vi "Main_SAIDD-Steffen’s MacBook Pro.vi"() -> ()   [LabVIEW 2018]
uses:
  <extravilib>/ChannelInstances/Tag-bool/Read With Abort.vi
  <extravilib>/ChannelInstances/Tag-bool/Write With Abort.vi
  <vilib>/myRIO/Common/Instrument Driver Framework/myRIO v1.0/UART/vis/myRIO v1.0 Close UART.vi
  <vilib>/Utility/error.llb/Error Cluster From Error Code.vi
  <vilib>/myRIO/Common/Instrument Driver Framework/myRIO v1.0/PWM/vis/myRIO v1.0 Write PWM.vi
  <vilib>/myRIO/Common/Instrument Driver Framework/myRIO v1.0/DIO/vis/myRIO v1.0 Write DIO.vi
  <extravilib>/ChannelInstances/Tag-bool/Instantiate.vi
  <extravilib>/ChannelInstances/Tag-bool/EndpointRead.vi
  <extravilib>/ChannelInstances/Tag-bool/Endpoint.vi
  <vilib>/myRIO/Common/Instrument Driver Framework/Utilities/vis/FPGA Ref Manager.vi
  <vilib>/myRIO/Common/Instrument Driver Framework/myRIO v1.0/myRIO v1.0 Reset FPGA.vi
  <vilib>/myRIO/Common/Instrument Driver Framework/myRIO v1.0/IRQ/vis/myRIO v1.0 IRQ Info FGV.vi
  <vilib>/myRIO/Common/Instrument Driver Framework/myRIO v1.0/IRQ/vis/myRIO v1.0 Timer IRQ Info FGV.vi
  <vilib>/myRIO/Common/Instrument Driver Framework/myRIO v1.0/IRQ/vis/myRIO v1.0 ISR Agent.vi
  <extravilib>/ChannelInstances/Tag-bool.lvlib
  <vilib>/myRIO/Instrument Drivers/Onboard IO/DIO/DIO.lvlib
  <vilib>/myRIO/Instrument Drivers/Onboard IO/PWM/PWM.lvlib
  <vilib>/myRIO/Instrument Drivers/Utilities/Utilities.lvlib
panel:
  in  "Beacon - test":bool
  in  "Grounded threshold":dbl=1.7 format="%#_13g"
  in  "QR - test":bool
  in  "Enable Triangle Wobble":bool=TRUE
  in  "Antal iterationer pr. stepper":i32=800
  in  "Stop":bool
  out "Measured current":dbl
  out "Ammeter measurement":dbl(graph)
  out "Duty Cycle":dbl
  out "Mean 200":dbl format="%0.2f"
  out "Battery left (%)":dbl
  in  "Drill - Frequency [Hz]":dbl=200.0
  in  "Stepper frekvens ned":dbl=120.0
  in  "Ingen modstand ned upper threshold":dbl=2750.0
  out "ALL TOP":bool
  out "ALL BOTTOM":bool
  in  "Resistance - Threshold Upper":dbl=3100.0
  in  "Resistance Threshold Lower":dbl=3025.0
  out "Process":T1(ring)
  in  "State":T1(ring)
  in  "high cutoff freq: fh":dbl=900.0
  in  "Radius":dbl=0.005 format="%#_13g"
  in  "Filter?":bool=TRUE
  out "RollDetection - Alarm":bool
types:
  T1 = enum16{"State 0 - Default", "State 1 - Go down", "State 2 - Go up", "State 3 - Triangle Wobble"}
  T2 = typedef "DIO.lvlib/DIO Reference.ctl" = cluster{"myRIO Reference":T3, "DIO Channels List":T7}
  T3 = typedef "myRIO Generic Hardware Reference.ctl" = cluster{"myRIO Model":T4, "myRIO Hardware Reference":T5}
  T4 = typedef "Hardware Version Enum.ctl" = enum16{"Unknown", "myRIO-1900", "myRIO-1950", "roboRIO", "NI ELVIS RIO CM", "ELVIS III"}
  T5 = typedef "myRIO v1.0 Reference.ctl" = cluster{"Generic FPGA Reference":T6, "Allow multiple opens":bool}
  T6 = typedef "Generic FPGA Reference.ctl" = refnum<k20>
  T7 = typedef "DIO Channels List.ctl" = T8[]
  T8 = typedef "DIO Channels Enum.ctl" = enum16{"Not Connected", "C/DIO0", "C/DIO1", "C/DIO2", "C/DIO3", "C/DIO4", "C/DIO5", "C/DIO6", "C/DIO7", "A/DIO0", "A/DIO1", "A/DIO2", "A/DIO3", "A/DIO4", "A/DIO5", "A/DIO6", "A/DIO7", "A/DIO8", "A/DIO9", "A/DIO10", "A/DIO11", "A/DIO12", "A/DIO13", "A/DIO14", "A/DIO15", "A/DIO16", "A/DIO17", "A/DIO18", "A/DIO19", "B/DIO0", "B/DIO1", "B/DIO2", "B/DIO3", "B/DIO4", "B/DIO5", "B/DIO6", "B/DIO7", "B/DIO8", "B/DIO9", "B/DIO10", "B/DIO11", "B/DIO12", "B/DIO13", "B/DIO14", "B/DIO15", "B/DIO16", "B/DIO17", "B/DIO18", "B/DIO19", "LED0", "LED1", "LED2", "LED3", "Button0", "DIO/DIO0", "DIO/DIO1", "DIO/DIO2", "DIO/DIO3", "DIO/DIO4", "DIO/DIO5", "DIO/DIO6", "DIO/DIO7", "DIO/DIO8", "DIO/DIO9", "SPI/CS0", "SPI/CS1", "SPI/CS2", "SPI/CS3", "LED RADIO (Green)", "LED RADIO (Red)", "LED COMM (Green)", "LED COMM (Red)", "LED MODE (Green)", "LED MODE (Red)"}
  T9 = typedef "PWM.lvlib/PWM Reference.ctl" = cluster{"myRIO Reference":T3, "PWM Channels Enum":T10, "PWM Configuration":T11}
  T10 = typedef "PWM Channels Enum.ctl" = enum16{"Not Connected", "C/PWM0", "C/PWM1", "A/PWM0", "A/PWM1", "A/PWM2", "A/PWM3", "A/PWM4", "A/PWM5", "A/PWM6", "A/PWM7", "A/PWM8", "A/PWM9", "A/PWM10", "A/PWM11", "A/PWM12", "A/PWM13", "A/PWM14", "A/PWM15", "A/PWM16", "A/PWM17", "A/PWM18", "A/PWM19", "B/PWM0", "B/PWM1", "B/PWM2", "B/PWM3", "B/PWM4", "B/PWM5", "B/PWM6", "B/PWM7", "B/PWM8", "B/PWM9", "B/PWM10", "B/PWM11", "B/PWM12", "B/PWM13", "B/PWM14", "B/PWM15", "B/PWM16", "B/PWM17", "B/PWM18", "B/PWM19", "PWM/PWM0", "PWM/PWM1", "PWM/PWM2", "PWM/PWM3", "PWM/PWM4", "PWM/PWM5", "PWM/PWM6", "PWM/PWM7", "PWM/PWM8", "PWM/PWM9"}
  T11 = typedef "PWM.lvlib/PWM Configuration.ctl" = cluster{"Frequency":dbl, "Duty Cycle":dbl}
  T12 = typedef "Accelerometer.lvlib/Accelerometer Reference.ctl" = cluster{"myRIO Reference":T3, "Accelerometer Channels List":T13, "LSB Weight":dbl}
  T13 = typedef "Accelerometer Channels List.ctl" = T14[]
  T14 = typedef "Accelerometer Channels Enum.ctl" = enum16{"Not Connected", "X-Axis", "Y-Axis", "Z-Axis"}
  T15 = typedef "AI.lvlib/AI Reference.ctl" = cluster{"myRIO Reference":T3, "AI Channels List":T16, "AI Scaling Constants List":T18}
  T16 = typedef "AI Channels List.ctl" = T17[]
  T17 = typedef "AI Channels Enum.ctl" = enum16{"Not Connected", "AudioIn/Left", "AudioIn/Right", "C/AI0", "C/AI1", "A/AI0", "A/AI1", "A/AI2", "A/AI3", "A/AI4", "A/AI5", "A/AI6", "A/AI7", "B/AI0", "B/AI1", "B/AI2", "B/AI3", "B/AI4", "B/AI5", "B/AI6", "B/AI7", "AI/AI0", "AI/AI1", "AI/AI2", "AI/AI3", "A/AI0 (DIFF)", "A/AI1 (DIFF)", "A/AI2 (DIFF)", "A/AI3 (DIFF)", "B/AI0 (DIFF)", "B/AI1 (DIFF)", "B/AI2 (DIFF)", "B/AI3 (DIFF)"}
  T18 = typedef "Analog Scaling Constants List.ctl" = T19[]
  T19 = typedef "Analog Scaling Constants.ctl" = cluster{"LSB Weight (Volts)":dbl, "Offset (Volts)":dbl, "Signed?":bool}
  T20 = typedef "SPI.lvlib/SPI Reference.ctl" = cluster{"myRIO Reference":T3, "SPI Channels Enum":T21, "SPI Configuration":T22}
  T21 = typedef "SPI Channels Enum.ctl" = enum16{"Not Connected", "A/SPI", "B/SPI", "SPI/SPI"}
  T22 = typedef "SPI.lvlib/SPI Configuration.ctl" = cluster{"Frequency [Hz]":dbl, "Clock Phase":T23, "Clock Polarity":T24, "Data Direction":T25, "Frame Length":T26}
  T23 = typedef "SPI Clock Phase.ctl" = enum8{"Leading", "Trailing"}
  T24 = typedef "SPI Clock Polarity.ctl" = enum8{"Low", "High"}
  T25 = typedef "SPI Data Direction.ctl" = enum8{"Most significant bit first", "Least significant bit first"}
  T26 = typedef "SPI Frame Length.ctl" = u8
  T27 = cluster{"B/DIO0 - Stepper Direction":T2, "B/DIO1 - Stepper1 Enable":T2, "B/DIO2 - Stepper2 Enable":T2, "B/DIO3 - Stepper3 Enable":T2, "B/DIO4 - Endstop Stepper1 Top":T2, "B/DIO11 - Endstop Stepper1 Bund":T2, "B/DIO12 - Endstop Stepper2 Top":T2, "B/DIO13 - Endstop Stepper2 Bund":T2, "B/DIO14 - Endstop Stepper3 Top":T2, "B/DIO15 - Endstop Stepper3 Bund":T2, "Deleted - A/DIO0 - Cooler":T2, "A/DIO1 - Beacon drop (dio1)":T2, "A/DIO2 - Beacon drop (dio0)":T2, "A/DIO3 - QuickRelease (dio1)":T2, "A/DIO4 - QuickRelease (dio0)":T2, "Deleted - A/DIO11 - LiDAR SPI CS":T2, "B/PWM0 - Stepper":T9, "B/PWM1 - Drill":T9, "Deleted - A/PWM0 - Servo_Roll":T9, "Deleted - A/PWM1 - Servo_Yaw":T9, "Acc. X-axis":T12, "Acc. Y-axis":T12, "B/AI0 - Drone Grounded S1 - F3":T15, "A/AI0 - QuickRelease S4 - F4":T15, "B/AI2 - Beacon Drop S5 - F5":T15, "B/AI3 - Begin drilling S3 - F6":T15, "B/AI1 - Gimbal Seach S8 - F8":T15, "Deleted - A/AI1 - Beacon Wiper":T15, "A/AI2 - QuickRelease Wiper":T15, "A/AI3 - Drill Current":T15, "Deleted - A/SPI - LiDAR":T20, "B/UART - XBee":refnum<visa-resource-name>, "Deleted - A/UART - A3 GPS":refnum<visa-resource-name>, "RIO Flashing LEDs":T2}
  T28 = typedef "Tag-bool.lvlib/))Channel.ctl" = refnum<queue>
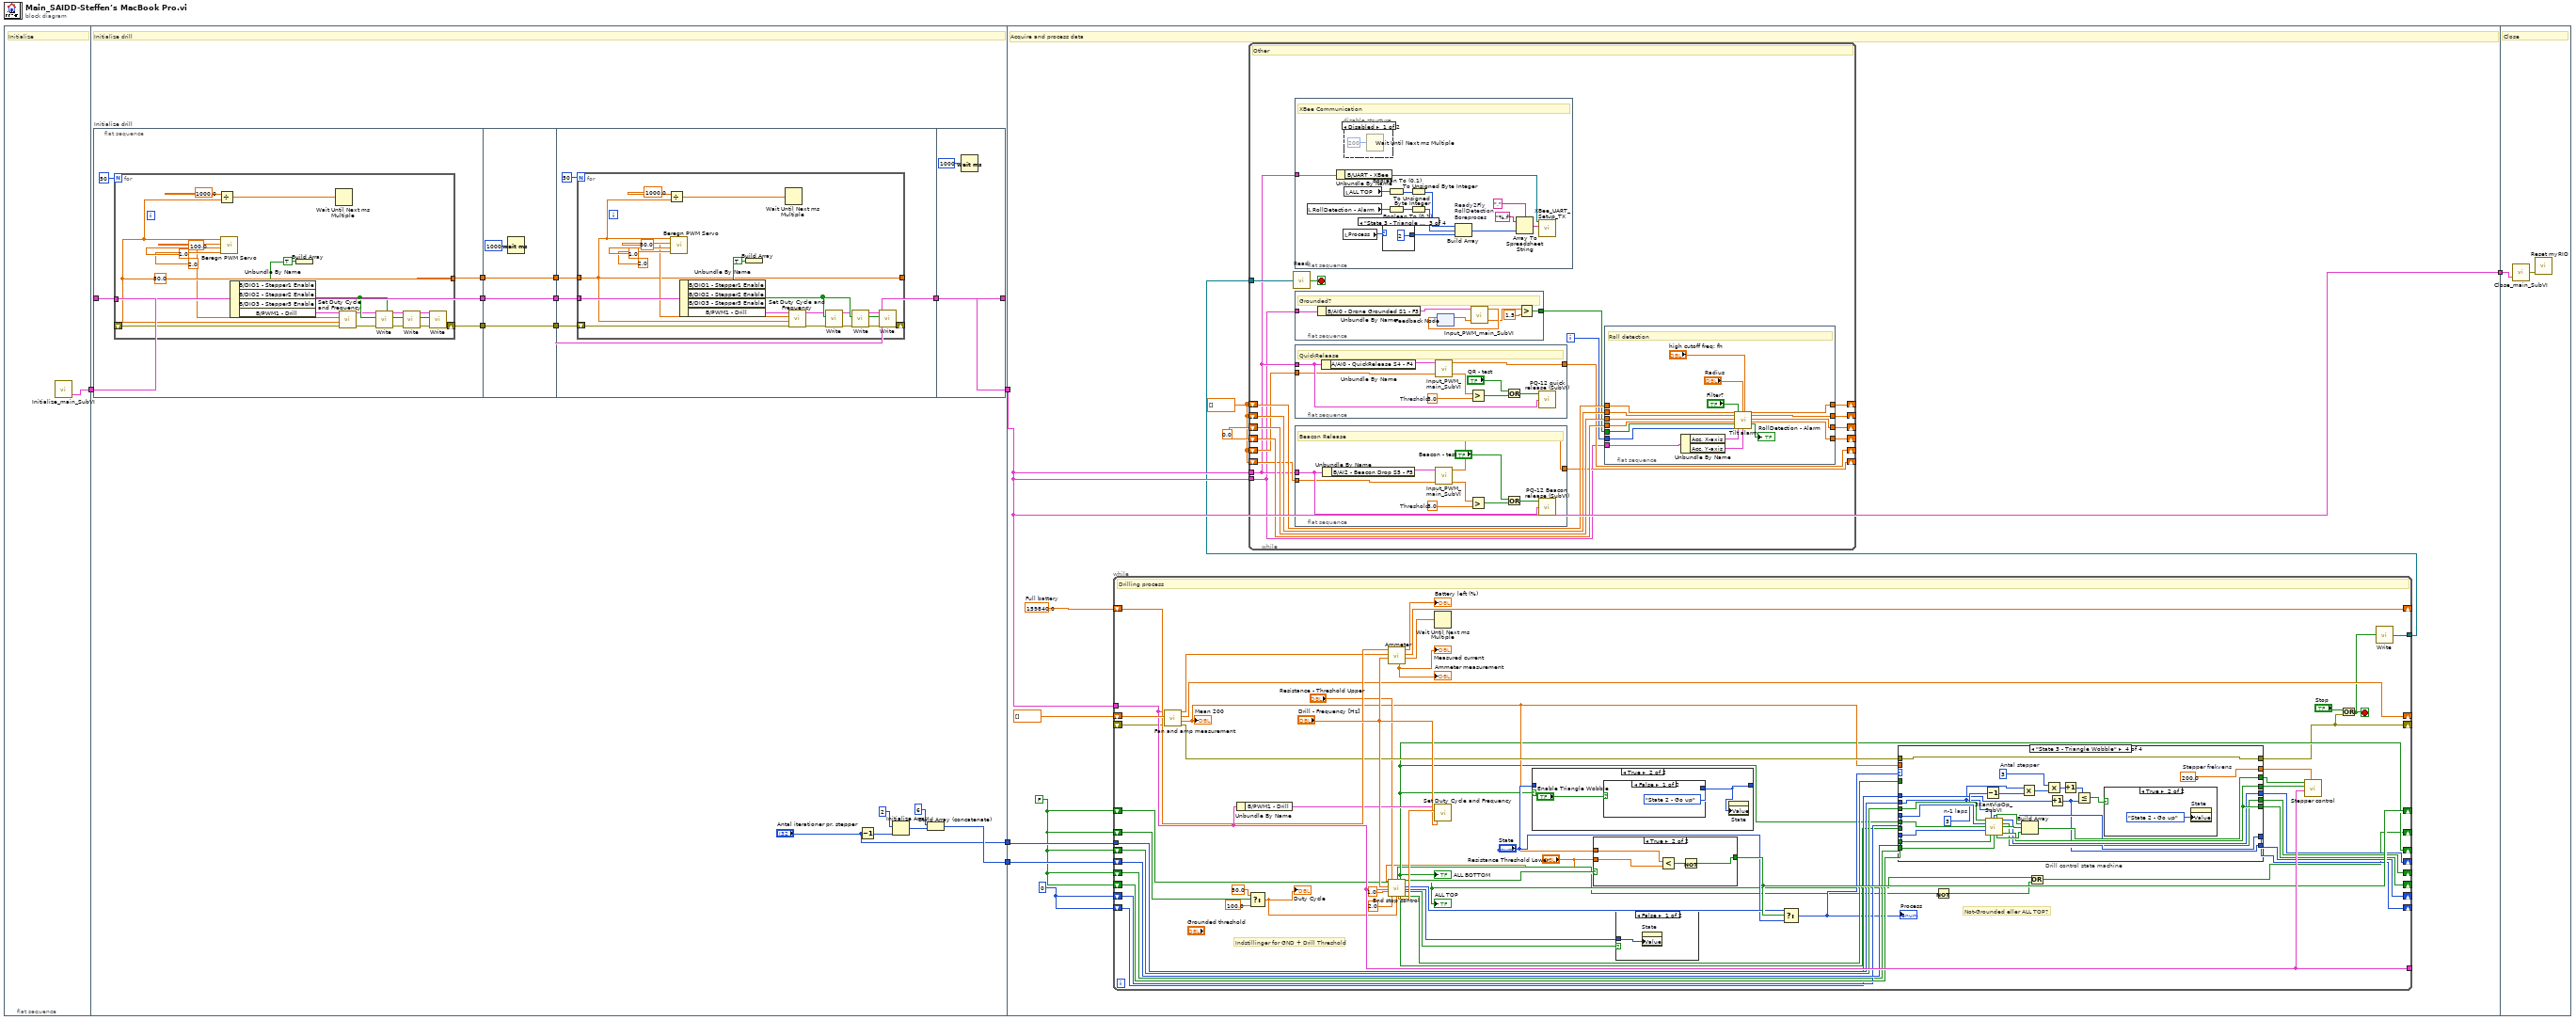
[diagram p0: block diagram]
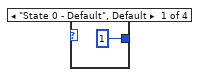
[diagram p3: hidden frame]
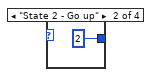
[diagram p4: hidden frame]
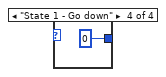
[diagram p5: hidden frame]
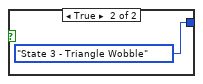
[diagram p8: hidden frame]
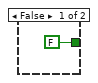
[diagram p9: hidden frame]
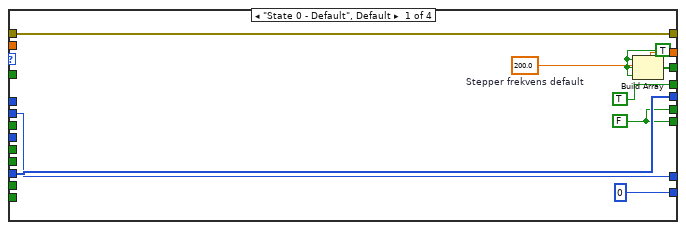
[diagram p10: hidden frame]
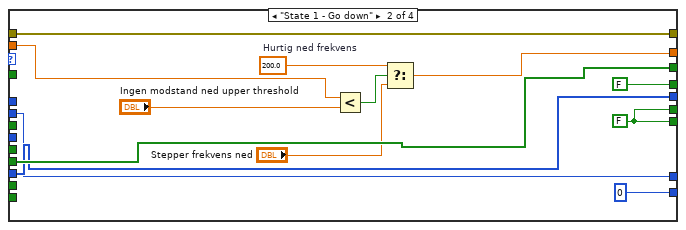
[diagram p11: hidden frame]
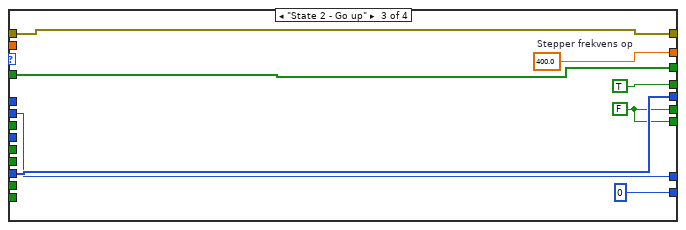
[diagram p12: hidden frame]
diagram:
  n1 = flat-sequence {
    tunnel: [w6] -> w4
    tunnel: w4 -> [w21]
    tunnel: [w18] -> w3
    tunnel: ["Antal iterationer pr. stepper"] -> w2
    tunnel: [w12] -> w1
    tunnel: w3 -> [w76]
    tunnel: [w76] -> w5
    tunnel: w2 -> [w79]
    tunnel: w1 -> [w78]
    tunnel: w5 -> [w289]
    frame #0 {
      # "Initialize"
      n2 = call "Initialize_main_SubVI.vi"() -> ("output cluster"=w6:T27)  [unwired: 2 in, 1 out]
    }
    frame #1 {
      # "Initialize drill"
      n3 = flat-sequence "Initialize drill" {
        tunnel: w21 -> [w25]
        tunnel: [w25] -> w20
        tunnel: [w24] -> w9
        tunnel: [w23] -> w7
        tunnel: w20 -> [w48]
        tunnel: [w48] -> w19
        tunnel: [w46] -> w10
        tunnel: w9 -> [w46]
        tunnel: [w45] -> w8
        tunnel: w7 -> [w45]
        tunnel: w19 -> [w52]
        tunnel: [w52] -> w17
        tunnel: w10 -> [w51]
        tunnel: w8 -> [w50]
        tunnel: [w73] -> w18
        tunnel: w17 -> [w73]
        frame #0 {
          n4 = for {
            N: 50 -> [_]
            tunnel: [w39] -> w24
            shift-right: [w32] -> w23
            shift-left: _ -> [w41]
            tunnel: w25 -> [w37]
            w39 = 50.0 ("Frequency [Hz]")
            n5 = Divide(x=1000.0, y=w39) -> (x/y=w40:dbl)
            n6 = call "Beregn PWM Servo.vi"("Max (ms puls bredde)"=2.0, "Min (ms puls bredde)"=1.0, "Duty Cycle"=100.0, "Frekvens"=w39) -> ("Output Dutycycle til PWM Servo"=w26:dbl)  [unwired: 7 in]
            n7 = Unbundle By Name(w37) -> ("B/DIO1 - Stepper1 Enable"=w27:T2, "B/DIO2 - Stepper2 Enable"=w28:T2, "B/DIO3 - Stepper3 Enable"=w29:T2, "B/PWM1 - Drill"=w31:T9)
            n8 = Build Array(TRUE) -> (w30:bool[])
            n9 = Wait Until Next ms Multiple(millisecond multiple=w40) -> ()  [unwired: 1 out]
            n10 = call <vilib>:"Set Duty Cycle and Frequency.vi"("error in (no error)"=w41, "Frequency [Hz]"=w39, "Duty Cycle"=w26, "PWM Ref In"=w31) -> ("error out"=w35:errorcluster)  [unwired: 5 in, 1 out]
            n11 = call <extravilib>:"Write.vi"("error in (no error)"=w35, "Values"=w30, "DIO Ref In"=w29) -> ("error out"=w34:errorcluster)  [unwired: 6 in, 1 out]
            n12 = call <extravilib>:"Write.vi"("error in (no error)"=w34, "Values"=w30, "DIO Ref In"=w28) -> ("error out"=w33:errorcluster)  [unwired: 6 in, 1 out]
            n13 = call <extravilib>:"Write.vi"("error in (no error)"=w33, "Values"=w30, "DIO Ref In"=w27) -> ("error out"=w32:errorcluster)  [unwired: 6 in, 1 out]
          }
        }
        frame #1 {
          n14 = Wait (ms)(milliseconds to wait=u32 1000) -> ()  [unwired: 1 out]
        }
        frame #2 {
          n15 = for {
            N: 50 -> [_]
            tunnel: [w53] -> _
            shift-right: [w60] -> _
            shift-left: w50 -> [w68]
            tunnel: w52 -> [w65]
            tunnel: w51 -> [w53]
            n16 = Divide(x=1000.0, y=w53) -> (x/y=w67:dbl)
            n17 = call "Beregn PWM Servo.vi"("Max (ms puls bredde)"=2.0, "Min (ms puls bredde)"=1.0, "Duty Cycle"=50.0, "Frekvens"=w53) -> ("Output Dutycycle til PWM Servo"=w54:dbl)  [unwired: 7 in]
            n18 = Unbundle By Name(w65) -> ("B/DIO1 - Stepper1 Enable"=w55:T2, "B/DIO2 - Stepper2 Enable"=w56:T2, "B/DIO3 - Stepper3 Enable"=w57:T2, "B/PWM1 - Drill"=w59:T9)
            n19 = Build Array(TRUE) -> (w58:bool[])
            n20 = Wait Until Next ms Multiple(millisecond multiple=w67) -> ()  [unwired: 1 out]
            n21 = call <vilib>:"Set Duty Cycle and Frequency.vi"("error in (no error)"=w68, "Frequency [Hz]"=w53, "Duty Cycle"=w54, "PWM Ref In"=w59) -> ("error out"=w63:errorcluster)  [unwired: 5 in, 1 out]
            n22 = call <extravilib>:"Write.vi"("error in (no error)"=w63, "Values"=w58, "DIO Ref In"=w57) -> ("error out"=w62:errorcluster)  [unwired: 6 in, 1 out]
            n23 = call <extravilib>:"Write.vi"("error in (no error)"=w62, "Values"=w58, "DIO Ref In"=w56) -> ("error out"=w61:errorcluster)  [unwired: 6 in, 1 out]
            n24 = call <extravilib>:"Write.vi"("error in (no error)"=w61, "Values"=w58, "DIO Ref In"=w55) -> ("error out"=w60:errorcluster)  [unwired: 6 in, 1 out]
          }
        }
        frame #3 {
          n25 = Wait (ms)(milliseconds to wait=u32 1000) -> ()  [unwired: 1 out]
        }
      }
      n26 = Decrement(x="Antal iterationer pr. stepper") -> (x-1=w16:i32)
      n27 = Initialize Array(2, w16) -> (w15:i32[])
      n28 = Build Array (concatenate)(6, w15) -> (w12:i32[])
    }
    frame #2 {
      w80 = 0.0 ("X-Stored-Shift-out")
      w81 = 0 ("Loops shift out")
      w77 = FALSE ("t")
      w83 = 159840.0  # Full battery
      w74 = dbl[] [] ("X-Array-Shift-out")
      # "Acquire and process data"
      n29 = while {
        shift-right: [w171] -> _
        shift-left: _ -> [w203]
        shift-right: [w175] -> _
        shift-left: dbl[] [] -> [w217]
        shift-right: [w213] -> _
        shift-left: w83 -> [w214]
        tunnel: w76 -> [w209]
        tunnel: [w209] -> _
        shift-right: [w205] -> _
        shift-left: w77 -> [w204]
        shift-right: [w168] -> _
        shift-left: w77 -> [w201]
        shift-right: [w199] -> _
        shift-left: w77 -> [w198]
        shift-right: [w197] -> _
        shift-left: w78 -> [w196]
        tunnel: w79 -> [w190]
        shift-right: [w194] -> _
        shift-left: w81 -> [w195]
        shift-right: [w193] -> _
        shift-left: w77 -> [w192]
        shift-right: [w173] -> _
        shift-left: w77 -> [w191]
        shift-right: [w188] -> _
        shift-left: w81 -> [w189]
        tunnel: [w164] -> w75
        stop <- w165 stop-if-true
        # "Not-Grounded eller ALL TOP?"
        # "Indstillinger for GND + Drill Threshold"
        # "Drilling process"
        n30 = call "Fan and amp measurement.vi"("error in (no error)"=w203, "Array in"=w217, "output cluster"=w209) -> ("error out"=w210:errorcluster, "Mean out"=w174:dbl, "Array out"=w175:dbl[], "dbl Scaled Value"=w207:dbl)  [unwired: 5 in]
        "Mean 200" <- w174
        n31 = Unbundle By Name(w209) -> ("B/PWM1 - Drill"=w211:T9)
        n32 = Select(t=50.0, s=w201, f=100.0 ("upper limit")) -> (s? t:f=w172:dbl)
        "Duty Cycle" <- w172
        n33 = call "Ammeter.vi"("Bor - Frequency [Hz]"="Drill - Frequency [Hz]", "Måling ammeter"=w207, "Sum batteri shift in"=w214) -> ("Wait ud"=w206:dbl, "Sum batteri shift ud"=w213:dbl, "Batteri tilbage (%)"=→"Battery left (%)":dbl, "Målt ampere"=→"Measured current" →"Ammeter measurement":dbl)  [unwired: 5 in]
        n34 = call "End stop control.vi"("Threshold Lower"="Resistance Threshold Lower", "t"=w204, "Bor - Frequency [Hz]"="Drill - Frequency [Hz]", "output cluster"=w209, "Min (ms puls bredde)"=1.0, "Threshold Upper"="Resistance - Threshold Upper", "Max (ms puls bredde)"=2.0, "Bor - Duty Cycle"=w172) -> ("Grounded?"=w166:bool, "Output Dutycycle \nPWM"=w216:dbl, "ALL BOTTOM"=w173:bool, "Bottom Array"=w185:bool[], "Boolean 2"=w182:bool, "ALL TOP"=w169:bool, "Enum 2"=w181:T1, "Enum"=w178:T1, "Boolean"=w179:bool, "Top Array"=w184:bool[])  [unwired: 8 in, 2 out]
        "ALL TOP" <- w169
        "ALL BOTTOM" <- w173
        n35 = Wait Until Next ms Multiple(millisecond multiple=w206) -> ()  [unwired: 1 out]
        n36 = call <vilib>:"Set Duty Cycle and Frequency.vi"("Frequency [Hz]"="Drill - Frequency [Hz]", "Duty Cycle"=w216, "PWM Ref In"=w211) -> ()  [unwired: 6 in, 2 out]
        n37 = case shown="True" w173 {
          tunnel: [w221 w222] -> _
          tunnel: "State" -> [w221 _]
          frame False {
          }
          frame True {
            n38 = case shown="False" "Enable Triangle Wobble" {
              tunnel: [T1."State 2 - Go up" ("Enum") T1."State 3 - Triangle Wobble" ("Enum")] -> w222
              frame False {
              }
              frame True {
              }
            }
            n39 = property on="State" class="Enum (strict)"("Value"=w222) -> ()  [unwired: 2 in, 2 out]
          }
        }
        n40 = case shown="True" w182 {
          tunnel: [FALSE w228] -> w205
          tunnel: w174 -> [_ w230]
          tunnel: "Resistance Threshold Lower" -> [_ w227]
          frame False {
          }
          frame True {
            n41 = Less?(x=w230, y=w227) -> (x < y?=w229:bool)
            n42 = Not(x=w229) -> (.not. x?=w228:bool)
          }
        }
        n43 = case shown="False" w179 {
          tunnel: w178 -> [w220 _]
          frame False {
            n44 = property on="State" class="Enum (strict)"("Value"=w220) -> ()  [unwired: 2 in, 2 out]
          }
          frame True {
          }
        }
        n45 = Select(t=w181, s=w205, f="State") -> (s? t:f=w177:T1)
        "Process" <- w177
        n46 = case "Drill control state machine" shown="\"State 3 - Triangle Wobble\"" w177 {
          tunnel: [w237 w252 w260 w281] -> w176
          tunnel: w185 -> [_ w252 _ _]
          tunnel: w184 -> [_ _ w260 _]
          tunnel: [TRUE FALSE TRUE w280] -> w208
          tunnel: w210 -> [w236 w250 w258 w285]
          tunnel: [w236 w250 w258 w285] -> w171
          tunnel: [w235 w247 w257 w286] -> w202
          tunnel: w174 -> [_ w244 _ _]
          tunnel: [w232 w241 w254 w280] -> w199
          tunnel: w198 -> [_ _ _ w279]
          tunnel: [w234 w243 w256 w278] -> w197
          tunnel: w196 -> [w234 w243 w256 w277]
          tunnel: w190 -> [w233 w242 w255 w267]
          tunnel: w195 -> [_ _ _ w276]
          tunnel: [w233 w242 w255 w275] -> w194
          tunnel: [w232 w241 w254 w274] -> w193
          tunnel: w192 -> [_ _ _ w273]
          tunnel: w191 -> [_ _ _ w272]
          tunnel: w173 -> [_ _ _ w270]
          tunnel: w189 -> [_ _ _ w269]
          tunnel: [0 0 0 w264] -> w188
          frame "State 0 - Default", Default {
            w232 = FALSE
            w235 = 200.0  # Stepper frekvens default
            w238 = TRUE
            n47 = Build Array(w238, w238, w238) -> (w237:bool[])
          }
          frame "State 1 - Go down" {
            w241 = FALSE
            w246 = 200.0  # Hurtig ned frekvens
            n48 = Less?(x=w244, y="Ingen modstand ned upper threshold") -> (x < y?=w249:bool)
            n49 = Select(t=w246, s=w249, f="Stepper frekvens ned") -> (s? t:f=w247:dbl)
          }
          frame "State 2 - Go up" {
            w254 = FALSE
            w257 = 400.0  # Stepper frekvens op
          }
          frame "State 3 - Triangle Wobble" {
            w265 = 3  # Antal stepper
            w271 = 3  # n-1 laps
            w286 = 200.0  # Stepper frekvens
            n50 = Decrement(x=w271) -> (x-1=w268:i32)
            n51 = call "3KantVipOp_SubVI.vi"("Shift 1 in"=w272, "Antal iterationer pr. stepper"=w267, "Loops shift in"=w276, "BUND!"=w270, "Index step array shift in"=w277, "Shift 2 in"=w273, "Shift 3 in"=w279) -> ("Loops shift out"=w275:i32, "Enable 1"=w282:bool, "Index step array shift ud"=w278:i32[], "Shift 2 ud"=w274:bool, "Enable 2"=w283:bool, "Enable 3"=w284:bool, "Direction"=w280:bool)  [unwired: 1 in, 1 out]
            n52 = Multiply(x=w267, y=w268) -> (x*y=w266:i32)
            n53 = Build Array(w282, w283, w284) -> (w281:bool[])
            n54 = Multiply(x=w265, y=w266) -> (x*y=w262:i32)
            n55 = Increment(x=w269) -> (x+1=w264:i32)
            n56 = Increment(x=w262) -> (x+1=w261:i32)
            n57 = Less Or Equal?(x=w261, y=w264) -> (x <= y?=w263:bool)
            n58 = case shown="True" w263 {
              frame False {
              }
              frame True {
                n59 = property on="State" class="Enum (strict)"("Value"=T1."State 2 - Go up" ("Enum")) -> ()  [unwired: 2 in, 2 out]
              }
            }
          }
        }
        n60 = Not(x=w166) -> (.not. x?=w167:bool)
        n61 = Or(x=w169, y=w167) -> (x .or. y?=w168:bool)
        n62 = call "Stepper control.vi"("Stepper frekvens"=w202, "output cluster"=w209, "Direction shift ud"=w208, "Array"=w176) -> ()  [unwired: 7 in, 1 out]
        n63 = Or(x="Stop", y=w171) -> (x .or. y?=w165:bool)
        n64 = call <extravilib>:"Write.vi"("element"=w165) -> ("channel"=w164:T28)  [unwired: 1 out]
      }
      n65 = while {
        shift-right: [w96] -> _
        shift-left: w74 -> [w101]
        shift-right: [w95] -> _
        shift-left: w74 -> [w100]
        shift-right: [w94] -> _
        shift-left: w80 -> [w99]
        shift-right: [w93] -> _
        shift-left: w80 -> [w98]
        tunnel: w75 -> [w92]
        tunnel: w76 -> [w84]
        tunnel: w76 -> [w86]
        shift-right: [w90] -> _
        shift-left: w74 -> [w89]
        shift-right: [w88] -> _
        shift-left: w74 -> [w87]
        i -> [w97]
        stop <- w91 stop-if-true
        # "Other"
        n66 = call <extravilib>:"Read.vi"("channel"=w92) -> ("element"=w91:bool)  [unwired: 1 in, 1 out]
        n67 = flat-sequence {
          tunnel: w86 -> [w122]
          frame #0 {
            # "XBee Communication"
            n68 = local read "RollDetection - Alarm"() -> (w111:bool)
            n69 = Unbundle By Name(w122) -> ("B/UART - XBee"=w121:refnum<visa-resource-name>)
            n70 = local read "Process"() -> (w116:T1)
            n71 = disable-structure shown="Disabled" {
              frame Disabled {
                n72 = Wait Until Next ms Multiple(millisecond multiple=u32 200) -> ()  [unwired: 1 out]
              }
              frame Enabled {
              }
            }
            n73 = local read "ALL TOP"() -> (w114:bool)
            n74 = case shown="\"State 3 - Triangle Wobble\"" w116 {
              tunnel: [u8 1 u8 2 u8 2 u8 0] -> w115
              frame "State 0 - Default", Default {
              }
              frame "State 2 - Go up" {
              }
              frame "State 3 - Triangle Wobble" {
              }
              frame "State 1 - Go down" {
              }
            }
            n75 = Boolean To (0,1)(Boolean=w114) -> (0, 1=w113:i16)
            n76 = Boolean To (0,1)(Boolean=w111) -> (0, 1=w110:i16)
            n77 = To Unsigned Byte Integer(number=w113) -> (unsigned 8bit integer=w112:u8)
            n78 = To Unsigned Byte Integer(number=w110) -> (unsigned 8bit integer=w109:u8)
            n79 = Build Array "Ready2Fly\nRollDetection\nBoreproces"(w112, w109, w115) -> (w117:u8[])
            n80 = Array To Spreadsheet String(delimiter (Tab)=",", array=w117, 3:"%.f" ("format string")) -> (spreadsheet string=w120:string)
            n81 = call "XBee_UART_Setup_TX.vi"("Characters to Write"=w120, "VISA resource name in"=w121) -> ()  [unwired: 9 in, 1 out]
          }
        }
        n82 = flat-sequence {
          tunnel: [w103] -> w85
          tunnel: w84 -> [w102]
          frame #0 {
            # "Grounded?"
            n83 = Unbundle By Name(w102) -> ("B/AI0 - Drone Grounded S1 - F3"=w104:T15)
            n84 = feedback #1() -> (w106:dbl[])  [unwired: 1 in]
            n85 = call "Input_PWM_main_SubVI.vi"("Shift in"=w106, "AI Ref In"=w104) -> ("Value out"=w105:dbl, "Shift out"=w107:dbl[])  [unwired: 1 in, 1 out]
            n86 = feedback-in #1(w107) -> ()
            n87 = Greater?(x=w105, y=1.5 ("x")) -> (0:w103:bool)
          }
        }
        n88 = flat-sequence {
          tunnel: w86 -> [w139]
          tunnel: [w138] -> w90
          tunnel: w89 -> [w137]
          frame #0 {
            w140 = 3.0  # Threshold
            # "QuickRelease"
            n89 = Unbundle By Name(w139) -> ("A/AI0 - QuickRelease S4 - F4"=w142:T15)
            n90 = call "Input_PWM_main_SubVI.vi"("Shift in"=w137, "AI Ref In"=w142) -> ("Value out"=w141:dbl, "Shift out"=w138:dbl[])  [unwired: 1 in, 1 out]
            n91 = Greater?(x=w141, y=w140) -> (0:w143:bool)
            n92 = Or(x="QR - test", y=w143) -> (x .or. y?=w144:bool)
            n93 = call "PQ-12 quick release (SubVI).vi"("output cluster"=w139, "Extend / Retract [F/T]"=w144) -> ()  [unwired: 1 in, 1 out]
          }
        }
        n94 = flat-sequence {
          tunnel: w86 -> [w131]
          tunnel: [w129] -> w88
          tunnel: w87 -> [w128]
          frame #0 {
            w136 = 3.0  # Threshold
            # "Beacon Release"
            n95 = Unbundle By Name(w131) -> ("B/AI2 - Beacon Drop S5 - F5"=w130:T15)
            n96 = call "Input_PWM_main_SubVI.vi"("Shift in"=w128, "AI Ref In"=w130) -> ("Value out"=w135:dbl, "Shift out"=w129:dbl[])  [unwired: 1 in, 1 out]
            n97 = Greater?(x=w135, y=w136) -> (0:w133:bool)
            n98 = Or(x="Beacon - test", y=w133) -> (x .or. y?=w134:bool)
            n99 = call "PQ-12 Beacon release (SubVI).vi"("output cluster"=w131, "Extend / Retract [T/F]"=w134) -> ()  [unwired: 1 in, 1 out]
          }
        }
        n100 = flat-sequence {
          tunnel: w101 -> [w162]
          tunnel: w100 -> [w161]
          tunnel: w99 -> [w160]
          tunnel: w98 -> [w159]
          tunnel: w97 -> [w158]
          tunnel: [w157] -> w96
          tunnel: [w156] -> w95
          tunnel: [w155] -> w94
          tunnel: [w154] -> w93
          tunnel: w85 -> [w152]
          tunnel: w84 -> [w146]
          frame #0 {
            # "Roll detection"
            n101 = Unbundle By Name(w146) -> ("Acc. X-axis"=w150:T12, "Acc. Y-axis"=w151:T12)
            n102 = call "Tilt alarm.vi"("X-Array-Shift-in"=w162, "Y-Array-Shift-in"=w161, "X-Stored-Shift-in"=w160, "Y-Stored-Shift-in"=w159, "Grounded?"=w152, "Iterations"=w158, "Filter?"="Filter?", "Accelerometer Ref X in"=w150, "Radius"="Radius", "Accelerometer Ref Y In"=w151, "high cutoff freq: fh"="high cutoff freq: fh") -> ("X-Array-Shift-out"=w157:dbl[], "Y-Array-Shift-out"=w156:dbl[], "X-Stored-Shift-out"=w155:dbl, "Y-Stored-Shift-out"=w154:dbl, "Alarm"=→"RollDetection - Alarm":bool)  [unwired: 11 in, 1 out]
          }
        }
      }
    }
    frame #3 {
      # "Close"
      n103 = call "Close_main_SubVI.vi"("output cluster"=w289) -> ("error out"=w288:errorcluster)  [unwired: 1 in]
      n104 = call <vilib>:"Reset myRIO.vi"("error in (no error)"=w288) -> ()  [unwired: 10 in, 1 out]
    }
  }
